vi "Leap Swipe Gesture Direction.vi"() -> ()   [LabVIEW 2011, in "LVH-Leap.lvlib"]
doc: "This example demonstrates how to read the direction (up, down, left, right, in, out) of a swipe gesture using the Leap Motion Controller."
uses:
  vi.lib/LabVIEW Hacker/Leap/LVH-Leap.lvlib
  vi.lib/LabVIEW Hacker/Leap/Public/Gestures/Swipe/Instance VIs/Read 1 Swipe Direction.vi
panel:
  out "Swipes":string
  in  "Stop Button":bool
  # "Leap Swipe Direction Example\n\nThis example demonstrates how to read the direction of a swipe gesture using the\n Leap Motion Controller.\n\nInstructions\n1. Connect the Leap Motion Controller to the host computer.\n2. Click the Run Arrow.\n3. Make a swipe gesture above the Leap and notice the swipe direction listed below."
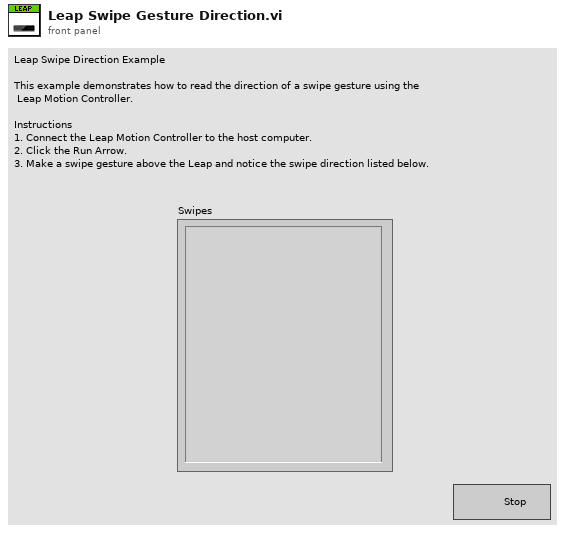
[diagram p1: front panel]
types:
  T1 = typedef "LVH-Leap.lvlib/Leap Handle.ctl" = cluster{"LeapCSharp":refnum<k24>}
  T2 = typedef "LVH-Leap.lvlib/Gesture State.ctl" = enum16{"Invalid", "Start", "Update", "Stop"}
  T3 = typedef "LVH-Leap.lvlib/Swipe Direction.ctl" = enum16{"Left", "Right", "Up", "Down", "In", "Out"}
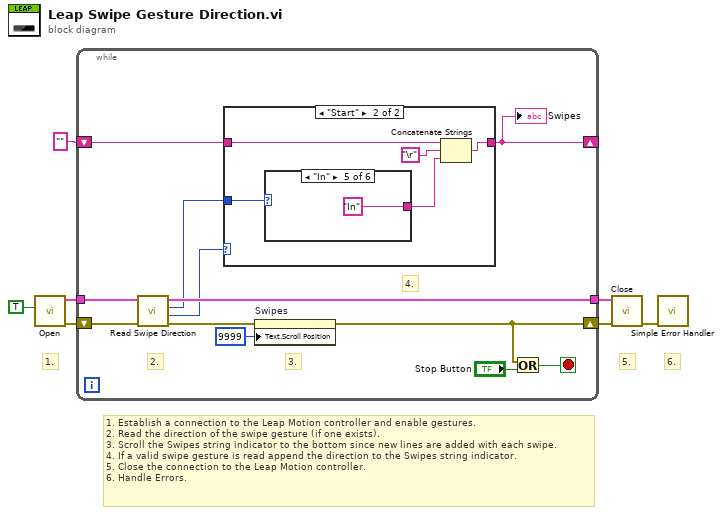
[diagram p0: block diagram]
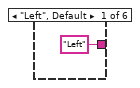
[diagram p3: hidden frame]
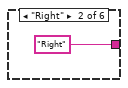
[diagram p4: hidden frame]
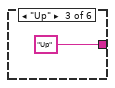
[diagram p5: hidden frame]
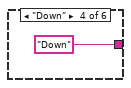
[diagram p6: hidden frame]
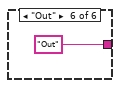
[diagram p7: hidden frame]
diagram:
  # "1. Establish a connection to the Leap Motion controller and enable gestures.\n2. Read the direction of the swipe gesture (if one exists).\n3. Scroll the Swipes string indicator to the bottom since new lines are added with each swipe.\n4. If a valid swipe gesture is read append the direction to the Swipes string indicator.\n5. Close the connection to the Leap Motion controller.\n6. Handle Errors."
  # "6."
  # "5."
  # "1."
  n1 = call "Open.vi"("Enable Gestures? (T)"=TRUE) -> ("Error Out"=w5:errorcluster, "Leap Handle"=w7:T1)  [unwired: 9 in]
  n2 = while {
    tunnel: w7 -> [w17]
    shift-right: [w9] -> w6
    shift-left: w5 -> [w15]
    tunnel: [w16] -> w3
    shift-right: [w12] -> _
    shift-left: "" -> [w11]
    stop <- w19 stop-if-true
    # "4."
    # "3."
    # "2."
    n3 = call-poly "Read Swipe Direction.vi"("Error In"=w15, "Leap Handle"=w17) -> ("Error Out"=w10:errorcluster, "Gesture State"=w13:T2, "Swipe Direction"=w14:T3, "Leap Handle"=w16:T1)  [unwired: 6 in]
    n4 = case shown="\"Start\"" w13 {
      tunnel: w14 -> [_ w25]
      tunnel: [w20 w24] -> w12
      tunnel: w11 -> [w20 w23]
      frame "Invalid", Default {
        # "No New Swipe"
      }
      frame "Start" {
        n5 = case shown="\"In\"" w25 {
          tunnel: ["Left" "Right" "Up" "Down" "In" "Out"] -> w21
          frame "Left", Default {
          }
          frame "Right" {
          }
          frame "Up" {
          }
          frame "Down" {
          }
          frame "In" {
          }
          frame "Out" {
          }
        }
        n6 = Concatenate Strings(w23, "\r", w21) -> (w24:string)
      }
    }
    "Swipes" <- w12
    n7 = property on="Swipes" class="Str"(error in=w10, "Text.Scroll Position"=u32 9999) -> (error out=w9:errorcluster)  [unwired: 1 in, 1 out]
    n8 = Or(x=w9, y="Stop Button") -> (x .or. y?=w19:bool)
  }
  n9 = call "Close.vi"("Error In"=w6, "Leap Handle"=w3) -> ("Error Out"=w2:errorcluster)  [unwired: 9 in]
  n10 = call <vilib>:"Simple Error Handler.vi"("error in (no error)"=w2) -> ()  [unwired: 4 in, 5 out]
